vi "Create WayPoints Approach CV crash.vi"(11 "input cluster":T2) -> (0 "output cluster":T1)   [LabVIEW 2023]
uses:
  TypeDefs/WayPointCluster.ctl
panel:
  in  "WayPointCluster":T1
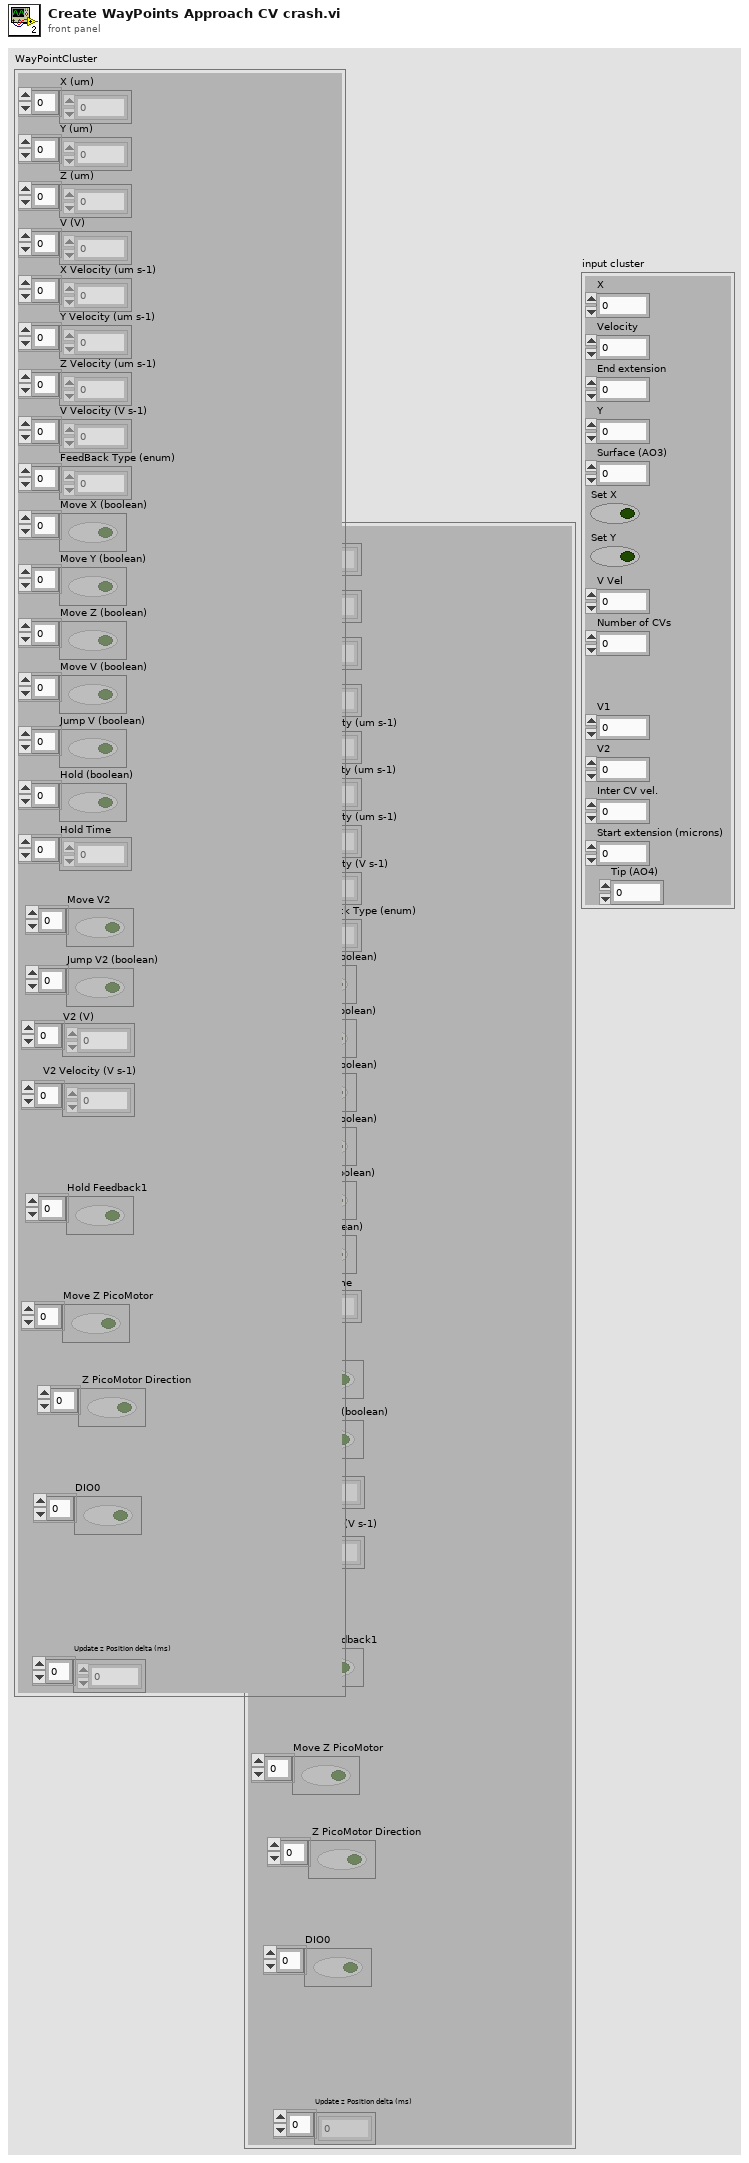
[diagram p1: front panel]
types:
  T1 = typedef "WayPointCluster.ctl" = cluster{"X (um)":dbl[], "Y (um)":dbl[], "Z (um)":dbl[], "V (V)":dbl[], "X Velocity (um s-1)":dbl[], "Y Velocity (um s-1)":dbl[], "Z Velocity (um s-1)":dbl[], "V Velocity (V s-1)":dbl[], "FeedBack Type (enum)":u16[], "Move X (boolean)":bool[], "Move Y (boolean)":bool[], "Move Z (boolean)":bool[], "Move V (boolean)":bool[], "Jump V (boolean)":bool[], "Hold (boolean)":bool[], "Hold Time":u32[], "V2 (V)":dbl[], "Move V2":bool[], "V2 Velocity (V s-1)":dbl[], "Jump V2 (boolean)":bool[], "Update z Position delta (ms)":i16[], "Hold Feedback1":bool[], "Move Z PicoMotor":bool[], " Z PicoMotor Direction":bool[], "DIO0":bool[]}
  T2 = cluster{"X":dbl, "Velocity":dbl, "End extension":dbl, "Y":dbl, "Surface (AO3)":dbl, "Set X":bool, "Set Y":bool, "V Vel":dbl, "Number of CVs":dbl, "V1":dbl, "V2":dbl, "Inter CV vel.":dbl, "Start extension (microns)":dbl, "Tip (AO4)":dbl}
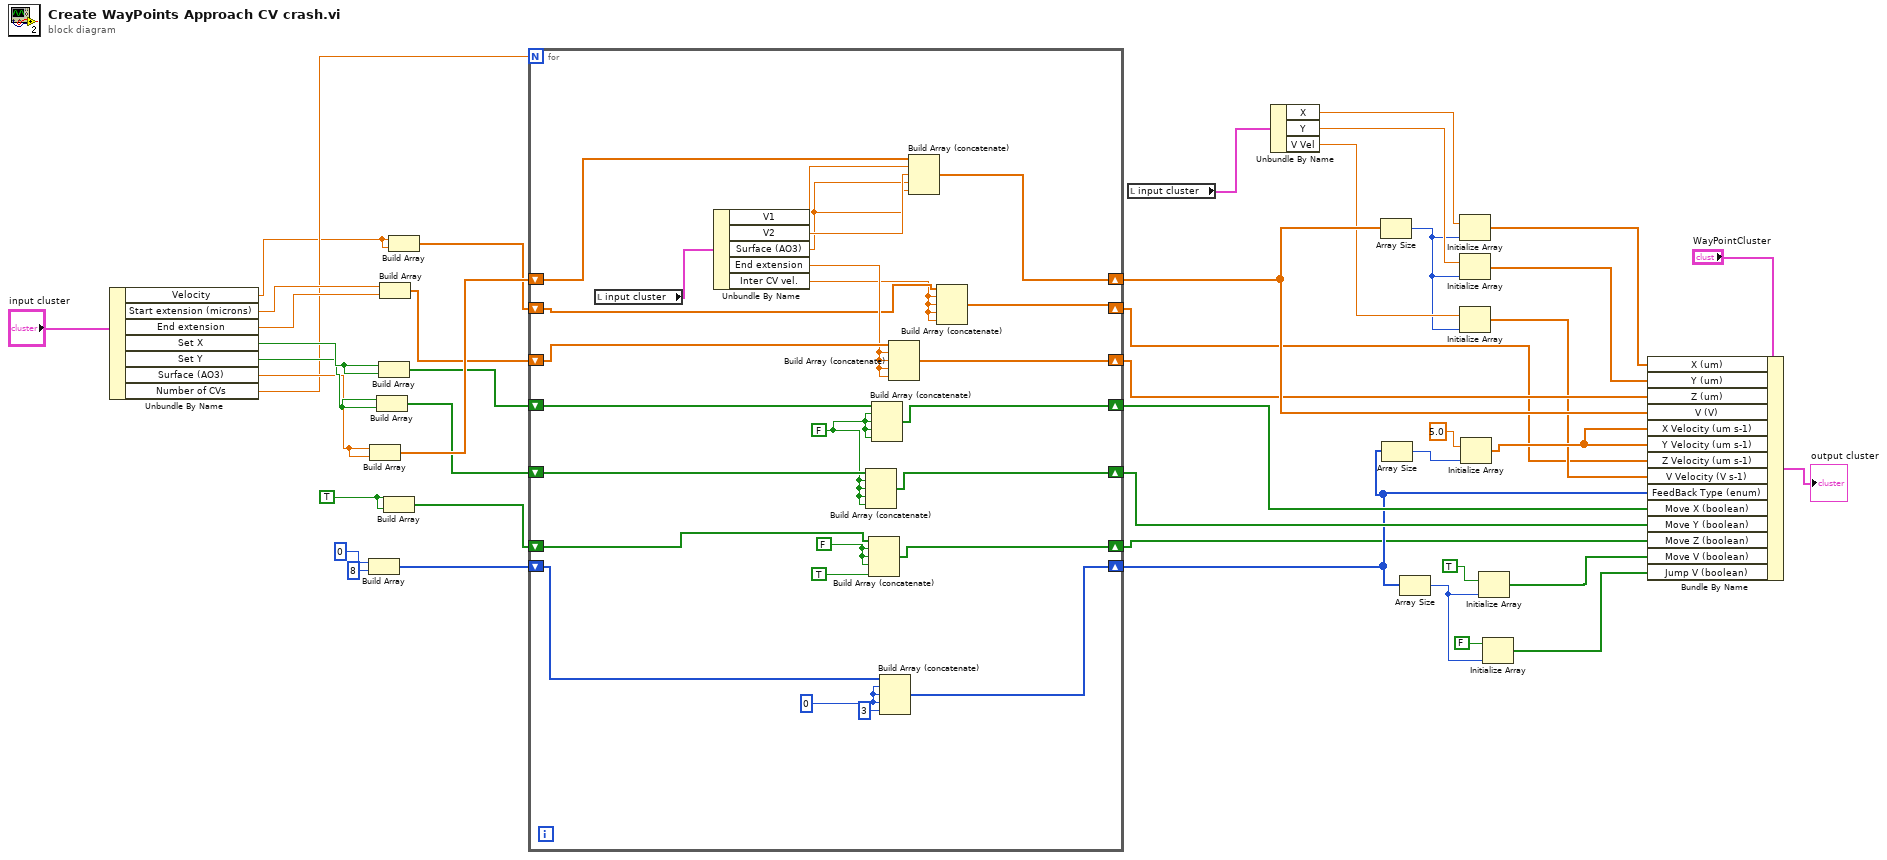
[diagram p0: block diagram]
diagram:
  w6 = TRUE
  n1 = Unbundle By Name("input cluster") -> ("Velocity"=w3:dbl, "Start extension (microns)"=w42:dbl, "End extension"=w41:dbl, "Set X"=w40:bool, "Set Y"=w39:bool, "Surface (AO3)"=w38:dbl, "Number of CVs"=w35:dbl)
  n2 = Build Array(i16 0 ("element"), i16 8 ("element")) -> (w32:i16[])
  n3 = Build Array(w38, w38) -> (w34:dbl[])
  n4 = Build Array(w39, w39) -> (w18:bool[])
  n5 = Build Array(w40, w40) -> (w19:bool[])
  n6 = Build Array(w42, w41) -> (w21:dbl[])
  n7 = Build Array(w6, w6) -> (w5:bool[])
  n8 = Build Array(w3, w3) -> (w2:dbl[])
  n9 = for {
    N: w35 -> [_]
    shift-right: [w64] -> w26
    shift-left: w34 -> [w63]
    shift-right: [w62] -> w14
    shift-left: w32 -> [w61]
    shift-right: [w58] -> w20
    shift-left: w21 -> [w57]
    shift-right: [w54] -> w17
    shift-left: w19 -> [w55]
    shift-right: [w51] -> w16
    shift-left: w18 -> [w53]
    shift-right: [w47] -> w4
    shift-left: w5 -> [w48]
    shift-right: [w46] -> w1
    shift-left: w2 -> [w45]
    w50 = FALSE
    w52 = FALSE
    w60 = i16 0 ("element")
    n10 = local read "input cluster"() -> (w68:T2)
    n11 = Unbundle By Name(w68) -> ("V1"=w67:dbl, "V2"=w66:dbl, "Surface (AO3)"=w65:dbl, "End extension"=w56:dbl, "Inter CV vel."=w44:dbl)
    n12 = Build Array (concatenate)(w53, w52, w52, w52, w52) -> (w51:bool[])
    n13 = Build Array (concatenate)(w48, w50, w50, w50, TRUE) -> (w47:bool[])
    n14 = Build Array (concatenate)(w55, w52, w52, w52, w52) -> (w54:bool[])
    n15 = Build Array (concatenate)(w61, w60, w60, w60, i16 3 ("element")) -> (w62:i16[])
    n16 = Build Array (concatenate)(w57, w56, w56, w56, w56) -> (w58:dbl[])
    n17 = Build Array (concatenate)(w63, w67, w66, w65, w65) -> (w64:dbl[])
    n18 = Build Array (concatenate)(w45, w44, w44, w44, w44) -> (w46:dbl[])
  }
  n19 = local read "input cluster"() -> (w27:T2)
  n20 = Unbundle By Name(w27) -> ("X"=w25:dbl, "Y"=w24:dbl, "V Vel"=w11:dbl)
  n21 = Array Size(array=w26) -> (size(s)=w9:i32)
  n22 = Array Size(array=w14) -> (size(s)=w15:i32)
  n23 = Array Size(array=w14) -> (size(s)=w7:i32)
  n24 = Initialize Array(w25, w9) -> (w23:dbl[])
  n25 = Initialize Array(w24, w9) -> (w22:dbl[])
  n26 = Initialize Array(w11, w9) -> (w10:dbl[])
  n27 = Initialize Array(5.0, w15) -> (w12:dbl[])
  n28 = Initialize Array(TRUE, w7) -> (w8:bool[])
  n29 = Initialize Array(FALSE, w7) -> (w28:bool[])
  n30 = Bundle By Name(cluster="WayPointCluster", "X (um)"=w23, "Y (um)"=w22, "Z (um)"=w20, "V (V)"=w26, "X Velocity (um s-1)"=w12, "Y Velocity (um s-1)"=w12, "Z Velocity (um s-1)"=w1, "V Velocity (V s-1)"=w10, "FeedBack Type (enum)"=w14, "Move X (boolean)"=w17, "Move Y (boolean)"=w16, "Move Z (boolean)"=w4, "Move V (boolean)"=w8, "Jump V (boolean)"=w28) -> (→"output cluster":T1)
